vi "Motion_Move Gantry and Check Position.vi"(5 "Timeout sec (-1 = No timeout)":i32=-1, 7 "Position Tolerance (0.1in)":dbl=0.1, 8 "error in":errorcluster, 10 "Gantry Move Data":T1={"Gantry Accel/Decel"=5.0, "Gantry Velocity"=5.0, "X-Position"=0.0, "Y-Position"=0.0, "Z-Position"=0.0} {"Z-Position" format="%_7g"; "Y-Position" format="%_7g"; "X-Position" format="%_7g"; "Gantry Velocity" format="%_7g"; "Gantry Accel/Decel" format="%_7g"}, 11 "TCP address:port":string="192.168.0.3:502") -> (0 "error out":errorcluster, 2 "elapsed time":dbl[unit]=nan format="%.1f", 3 "In Position?":bool)   [LabVIEW 2010]
uses:
  Motion_Gantry Position.ctl
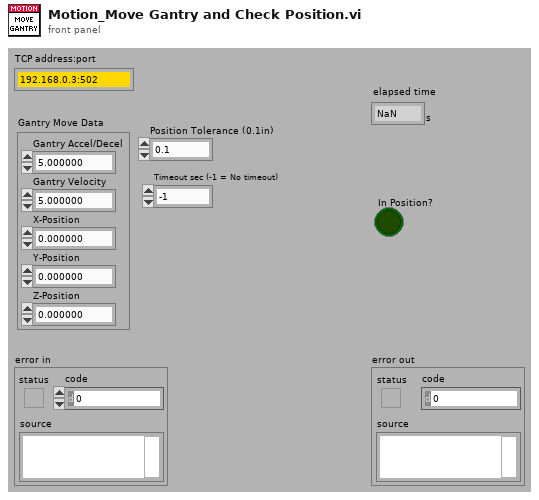
[diagram p1: front panel]
types:
  T1 = typedef "Motion_Gantry Position.ctl" = cluster{"Gantry Accel/Decel":dbl, "Gantry Velocity":dbl, "X-Position":dbl, "Y-Position":dbl, "Z-Position":dbl}
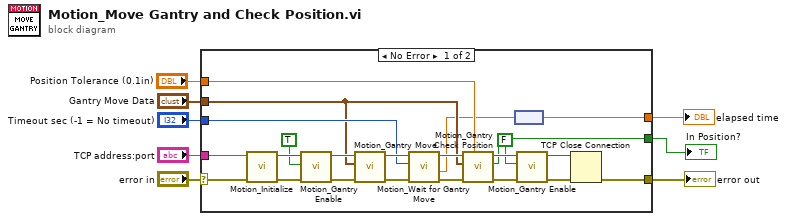
[diagram p0: block diagram]
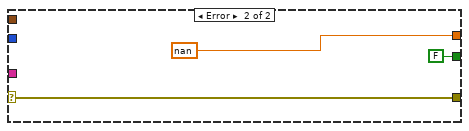
[diagram p2: hidden frame]
diagram:
  n1 = case shown="No Error" "error in" {
    selector: "error in" -> [w29 w34]
    tunnel: [w31 w34] -> w8
    tunnel: "TCP address:port" -> [w30 _]
    tunnel: [w10 dbl[unit] nan ("elapsed time")] -> w5
    tunnel: "Timeout sec (-1 = No timeout)" -> [w18 _]
    tunnel: "Gantry Move Data" -> [w17 _]
    tunnel: "Position Tolerance (0.1in)" -> [w12 _]
    tunnel: [w9 FALSE ("In Position?")] -> w1
    frame No Error {
      n2 = call "Motion_Initialize.vi"("error in"=w29, "TCP address:port (192.168.0.3:502)"=w30) -> ("error out"=w28:errorcluster, "connection ID"=w27:refnum<k5>)  [unwired: 8 in]
      n3 = call "Motion_Gantry Enable.vi"("error in (no error)"=w28, "Enable? (T)"=TRUE, "TCP Connection Refnum in"=w27) -> ("error out"=w25:errorcluster, "TCP Connection Refnum (dup)"=w26:refnum<k5>)  [unwired: 7 in]
      n4 = call "Motion_Gantry Move.vi"("error in (no error)"=w25, "Gantry Move Data"=w17, "TCP Connection Refnum in"=w26) -> ("error out"=w22:errorcluster, "TCP Connection Refnum (dup)"=w23:refnum<k5>)  [unwired: 7 in]
      n5 = call "Motion_Wait for Gantry Move.vi"("error in (no error)"=w22, "Timeout sec (-1 = No timeout)"=w18, "TCP Connection Refnum in"=w23) -> ("error out"=w20:errorcluster, "Time Elapsed"=w11:dbl, "TCP Connection Refnum (dup)"=w21:refnum<k5>)  [unwired: 5 in, 1 out]
      n6 = call "Motion_Gantry Check Position.vi"("Tolerance (0.1)"=w12, "error in (no error)"=w20, "Gantry Move Data"=w17, "TCP Connection Refnum"=w21) -> ("error out"=w15:errorcluster, "In Position?"=w9:bool, "TCP Connection Refnum (dup)"=w19:refnum<k5>)  [unwired: 5 in]
      n7 = node(w11) -> (w10:dbl[unit])
      n8 = call "Motion_Gantry Enable.vi"("error in (no error)"=w15, "Enable? (T)"=FALSE, "TCP Connection Refnum in"=w19) -> ("error out"=w13:errorcluster, "TCP Connection Refnum (dup)"=w14:refnum<k5>)  [unwired: 7 in]
      n9 = TCP Close Connection(connection ID=w14, error in (no error)=w13) -> (error out=w31:errorcluster)  [unwired: 1 in, 1 out]
    }
    frame Error {
    }
  }
  "error out" <- w8
  "elapsed time" <- w5
  "In Position?" <- w1
